vi "Visit.vi"(8 "error in (no error)":errorcluster, 10 "Equipment":refnum<class "Equipment.lvclass">, 11 "reference in":refnum<class "PrintVisitor.lvclass">) -> (0 "error out":errorcluster, 3 "reference in":refnum<class "PrintVisitor.lvclass">)   [LabVIEW 2012]
uses:
  PrintVisitor.lvclass
  Equipment_class/Equipment.lvclass
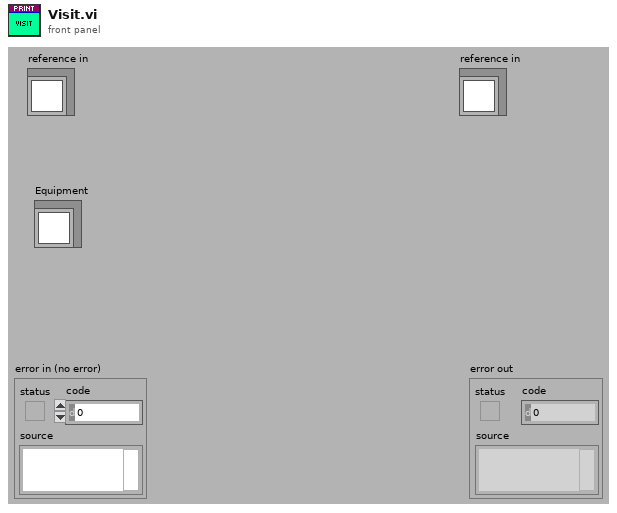
[diagram p1: front panel]
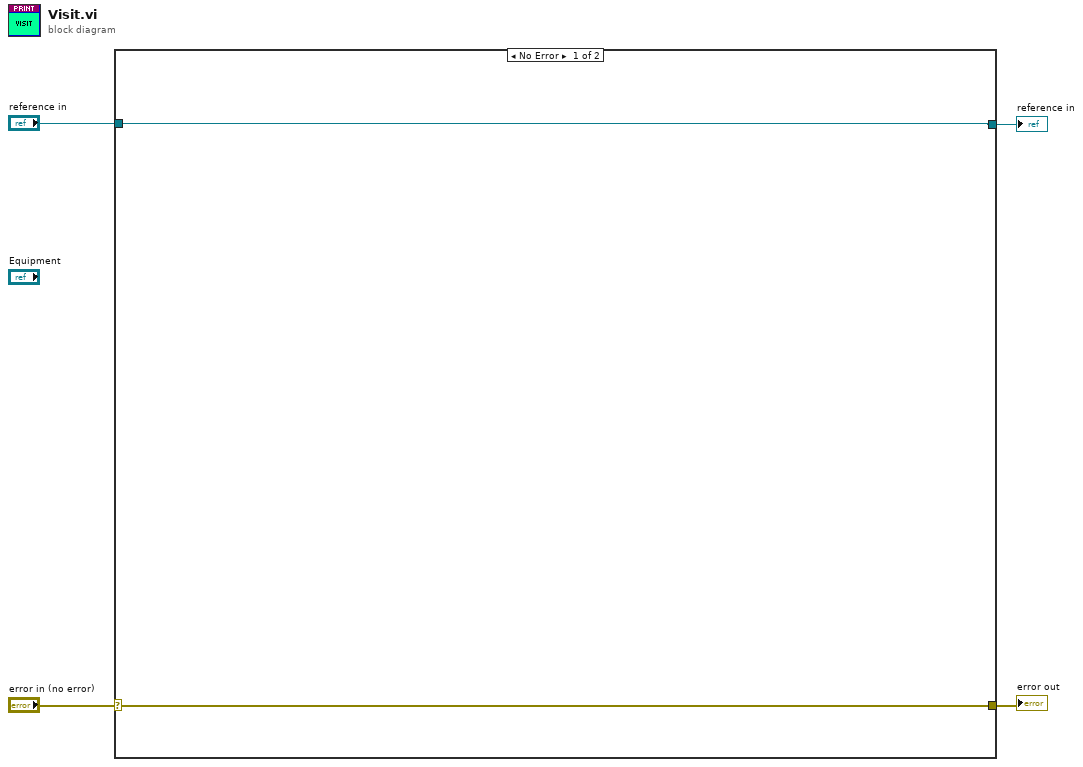
[diagram p0: block diagram]
diagram:
  n1 = case shown="No Error" "error in (no error)" {
    selector: "error in (no error)" -> [w5 w8]
    tunnel: [w5 w8] -> w3
    tunnel: [w6 w7] -> w1
    tunnel: "reference in" -> [w6 w7]
    frame No Error {
    }
    frame Error {
    }
  }
  "error out" <- w3
  "reference in" <- w1
